vi "Save Configuration Settings to XML.vi"(8 "error in (no error)":cluster{"状态":bool, "代码":i32, "源":string} caption="错误输入（无错误）", 11 "用户配置":T1={"硬件配置"={"硬件引用句柄<替换此项>"="", "信号类型<替换该项>"=enum."Sine Wave"}, "分析配置"={"统计"=TRUE}, "新采集到数据时如何操作"=enum."Replace"}) -> (0 "error out":cluster{"状态":bool, "代码":i32, "源":string} caption="错误输出")   [LabVIEW 2013]
doc: "将用户设定的配置数据保存至XML文件。本VI可在多次执行之间保持设置。"
uses:
  controls/User Specified Data.ctl
  controls/HW Configuration.ctl
  controls/Simulated Signal Type.ctl
  controls/Analysis Configuration.ctl
  controls/New Data Behavior.ctl
  <vilib>/Utility/xml.llb/Write to XML File(string).vi
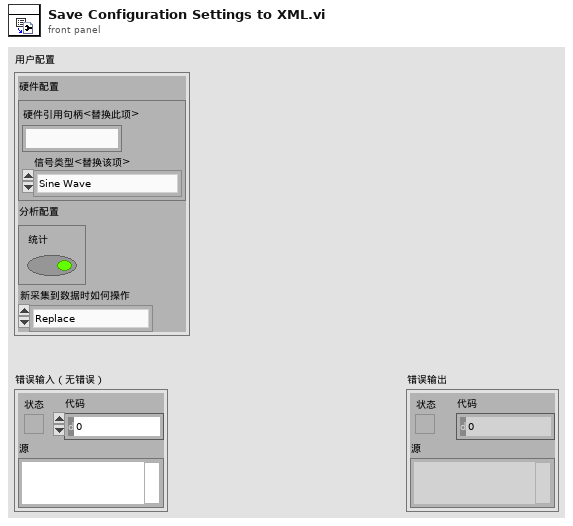
[diagram p1: front panel]
types:
  T1 = typedef "User Specified Data.ctl" = cluster{"硬件配置":T2, "分析配置":T4, "新采集到数据时如何操作":T5}
  T2 = typedef "HW Configuration.ctl" = cluster{"硬件引用句柄<替换此项>":string, "信号类型<替换该项>":T3}
  T3 = typedef "Simulated Signal Type.ctl" = enum16{"Sine Wave", "Square Wave"}
  T4 = typedef "Analysis Configuration.ctl" = cluster{"统计":bool}
  T5 = typedef "New Data Behavior.ctl" = enum16{"Replace", "Overlay", "Append"}
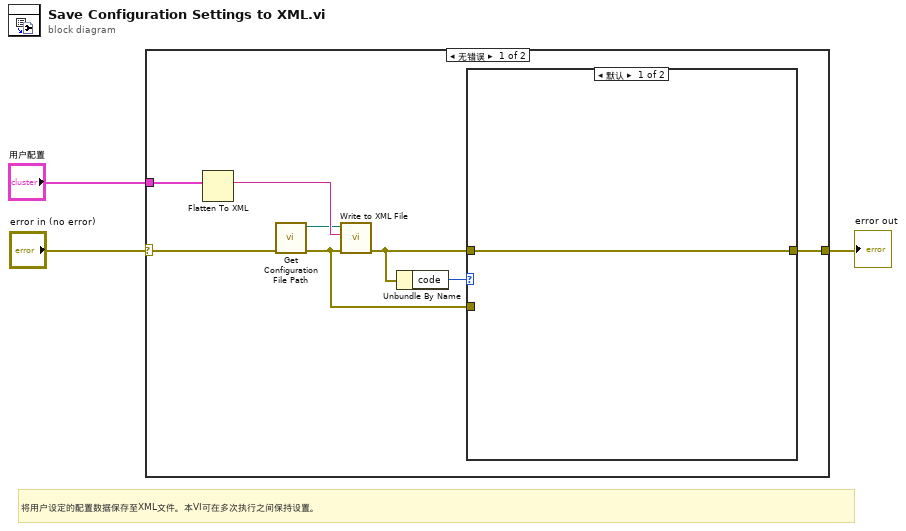
[diagram p0: block diagram]
diagram:
  # "将用户设定的配置数据保存至XML文件。本VI可在多次执行之间保持设置。"
  n1 = case shown="无错误" "error in (no error)" {
    selector: "error in (no error)" -> [w8 w14]
    tunnel: [w5 w14] -> w2
    tunnel: "用户配置" -> [w11 _]
    frame No Error {
      n2 = Flatten To XML(anything=w11) -> (xml string=w10:string)
      n3 = call "Get Configuration File Path.vi"("error in (no error)"=w8) -> ("error out"=w4:cluster{"状态":bool, "代码":i32, "源":string}, "XML文件路径"=w9:path)  [unwired: 9 in]
      n4 = call-poly <vilib>:"Write to XML File.vi"("error in (no error)"=w4, "XML Input"=w10, "XML File Path"=w9) -> ("error out"=w6:errorcluster)  [unwired: 6 in, 2 out]
      n5 = Unbundle By Name(w6) -> ("code"=w7:i32)
      n6 = case shown="默认" w7 {
        tunnel: [w12 w13] -> w5
        tunnel: w6 -> [w12 _]
        tunnel: w4 -> [_ w13]
        frame Default {
        }
        frame 8 {
          # "尝试保存Settings.xml文件时忽略权限错误。"
          # "#推荐代码 - 保存Settings.xml文件时可能出现权限错误，可在此处添加对权限错误执行额外处理的代码。"
        }
      }
    }
    frame Error {
    }
  }
  "error out" <- w2
